vi "write.vi"(8 "error in (no error)":errorcluster, 10 "String to send":string, 11 "EMTestCWS500N in":refnum<class "EMTestCWS500N.lvclass">) -> (0 "error out":errorcluster, 3 "EMTestCWS500N out":refnum<class "EMTestCWS500N.lvclass">)   [LabVIEW 2013, in "EMTestCWS500N.lvclass"]
uses:
  EMTestCWS500N.lvclass
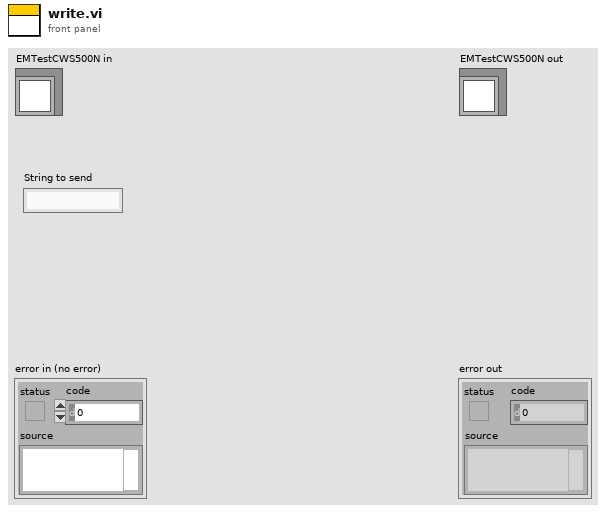
[diagram p1: front panel]
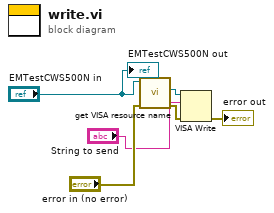
[diagram p0: block diagram]
diagram:
  n1 = call-dynamic "get VISA resource name.vi"("error in (no error)"="error in (no error)", "DeviceInterface (Eingang)"="EMTestCWS500N in") -> ("error out"=w2:errorcluster, "VISA resource name"=w5:refnum<visa-resource-name>)  [unwired: 7 in, 1 out]
  n2 = VISA Write(VISA resource name=w5, write buffer="String to send", error in (no error)=w2) -> (error out=→"error out":errorcluster)  [unwired: 2 out]
  "EMTestCWS500N out" <- "EMTestCWS500N in"
